vi "days_diff.vi"(3 "day":dbl=10.0, 4 "month":dbl=3.0, 5 "year":dbl=2013.0) -> (0 "New Date":timestamp, 1 "Days Diff":dbl, 2 "Current Date":timestamp)   [LabVIEW 2011]
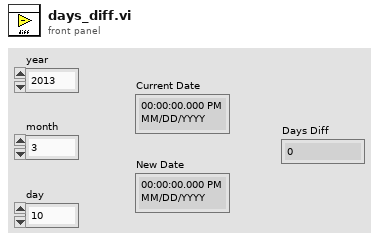
[diagram p1: front panel]
types:
  T1 = cluster{"second":i32, "minute":i32, "hour":i32, "day of month":i32, "month":i32, "year":i32, "day of week":i32, "day of year":i32, "is DST":i32}
  T2 = typedef "LVDateTimeRec.ctl" = cluster{"fractional second":dbl, "second":i32, "minute":i32, "hour":i32, "day of month":i32, "month":i32, "year":i32, "day of week":i32, "day of year":i32, "DST":i32}
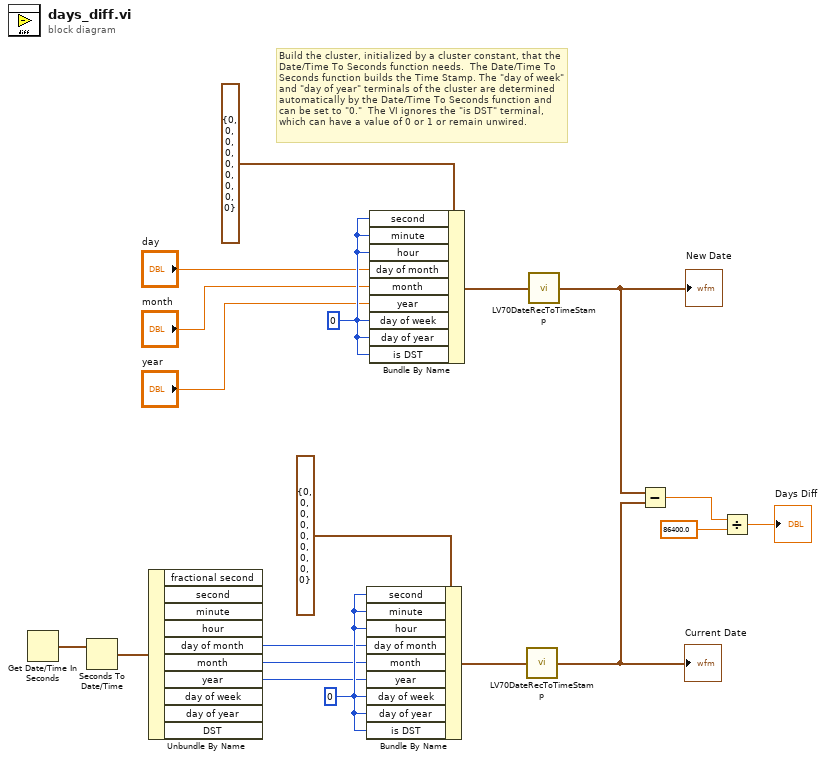
[diagram p0: block diagram]
diagram:
  w16 = 0
  w17 = 0
  # "Build the cluster, initialized by a cluster constant, that the Date/Time To Seconds function needs.  The Date/Time To Seconds function builds the Time Stamp. The \"day of week\" and \"day of year\" terminals of the cluster are determined automatically by the Date/Time To Seconds function and can be set to \"0.\"  The VI ignores the \"is DST\" terminal, which can have a value of 0 or 1 or remain unwired."
  n1 = Get Date/Time In Seconds() -> (seconds since 1Jan1904=w8:timestamp)
  n2 = Seconds To Date/Time(time stamp (now)=w8) -> (date time rec=w7:T2)  [unwired: 1 in]
  n3 = Unbundle By Name(w7) -> ("day of month"=w6:i32, "month"=w5:i32, "year"=w4:i32)  [unwired: 7 out]
  n4 = Bundle By Name(cluster=T1 {"second"=0, "minute"=0, "hour"=0, "day of month"=0, "month"=0, "year"=0, "day of week"=0, "day of year"=0, "is DST"=0} ("date time rec"), "second"=w17, "minute"=w17, "hour"=w17, "day of month"=w6, "month"=w5, "year"=w4, "day of week"=w17, "day of year"=w17, "is DST"=w17) -> (w18:T1)
  n5 = Bundle By Name(cluster=T1 {"second"=0, "minute"=0, "hour"=0, "day of month"=0, "month"=0, "year"=0, "day of week"=0, "day of year"=0, "is DST"=0} ("date time rec"), "second"=w16, "minute"=w16, "hour"=w16, "day of month"="day", "month"="month", "year"="year", "day of week"=w16, "day of year"=w16, "is DST"=w16) -> (w15:T1)
  n6 = call <vilib>:"LV70DateRecToTimeStamp.vi"("date time rec"=w18) -> ("Time Stamp"=w12:timestamp)
  "Current Date" <- w12
  n7 = call <vilib>:"LV70DateRecToTimeStamp.vi"("date time rec"=w15) -> ("Time Stamp"=w13:timestamp)
  "New Date" <- w13
  n8 = Subtract(x=w13, y=w12) -> (x-y=w11:dbl)
  n9 = Divide(x=w11, y=86400.0) -> (x/y=→"Days Diff":dbl)
